vi "Andor_Configuration.vi"(8 "Error in":errorcluster) -> (0 "error out":errorcluster, 3 "image":i32[][](array[numeric]))   [LabVIEW 2011]
uses:
  lib/atmcd32d.llb/ReadMode_mode typedef.ctl
  lib/atmcd32d.llb/AcquisitionMode_mode typedef.ctl
  lib/atmcd32d.llb/TriggerMode_mode typedef.ctl
  lib/atmcd32d.llb/Shutter_type typedef.ctl
  lib/atmcd32d.llb/Shutter_mode typedef.ctl
  lib/atmcd32d.llb/HSSpeed_type typedef.ctl
  lib/atmcd32d.llb/EMGainMode_mode typedef.ctl
  lib/atmcd32d.llb/Error Code Enum typedef.ctl
  Variables/GlobalSetGetConfigureCamera.vi
  Variables/ccdChipPixels.vi
panel:
  out "low":i32
  out "high":i32
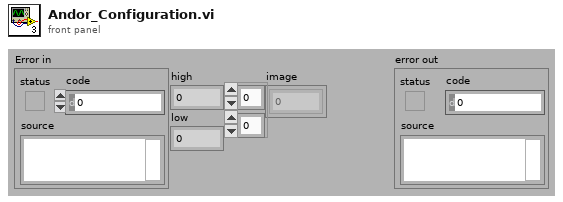
[diagram p1: front panel]
types:
  T1 = typedef "EMGainMode_mode typedef.ctl" = enum16{"8-bit", "12-bit", "Linear", "Real"}
  T2 = typedef "HSSpeed_type typedef.ctl" = enum16{"EM Amp", "Conventional Amp"}
  T3 = typedef "Shutter_mode typedef.ctl" = enum16{"Auto", "Open", "Close"}
  T4 = typedef "Shutter_type typedef.ctl" = enum16{"TTL Low", "TTL High"}
  T5 = typedef "TriggerMode_mode typedef.ctl" = enum16{"Internal", "External", "N/A (2)", "N/A (3)", "N/A (4)", "N/A (5)", "External Start"}
  T6 = typedef "AcquisitionMode_mode typedef.ctl" = enum16{"Reserved (0)", "Single Scan", "Accumulate", "Kinetics", "Fast Kinetics", "Run Till Abort", "Reserved (6)", "Reserved (7)", "Reserved (8)", "Time Delayed Integration"}
  T7 = typedef "ReadMode_mode typedef.ctl" = enum16{"Full Vertical Binning", "Multi-Track", "Random-Track", "Single-Track", "Image"}
  T8 = typedef "Error Code Enum typedef.ctl" = enum32{"N/A (0)", "DRV_ERROR_CODES", "DRV_SUCCESS", "DRV_VXDNOTINSTALLED", "DRV_ERROR_SCAN", "DRV_ERROR_CHECK_SUM", "DRV_ERROR_FILELOAD", "DRV_UNKNOWN_FUNC", "DRV_ERROR_VXD_INIT", "DRV_ERROR_ADDRESS", "DRV_ERROR_PAGELOCK", "DRV_ERROR_PAGEUNLOCK", "DRV_ERROR_BOARDTEST", "DRV_ERROR_ACK", "DRV_ERROR_UP_FIFO", "DRV_ERROR_PATTERN", "N/A (16)", "DRV_ACQUISITION_ERRORS", "DRV_ACQ_BUFFER", "DRV_ACQ_DOWNFIFO_FULL", "DRV_PROC_UNKONWN_INSTRUCTION", "DRV_ILLEGAL_OP_CODE", "DRV_KINETIC_TIME_NOT_MET", "DRV_ACCUM_TIME_NOT_MET", "DRV_NO_NEW_DATA", "N/A (25)", "DRV_SPOOLERROR", "N/A (27)", "N/A (28)", "N/A (29)", "N/A (30)", "N/A (31)", "N/A (32)", "DRV_TEMPERATURE_CODES", "DRV_TEMPERATURE_OFF", "DRV_TEMPERATURE_NOT_STABILIZED", "DRV_TEMPERATURE_STABILIZED", "DRV_TEMPERATURE_NOT_REACHED", "DRV_TEMPERATURE_OUT_RANGE", "DRV_TEMPERATURE_NOT_SUPPORTED", "DRV_TEMPERATURE_DRIFT", "N/A (41)", "N/A (42)", "N/A (43)", "N/A (44)", "N/A (45)", "N/A (46)", "N/A (47)", "N/A (48)", "DRV_GENERAL_ERRORS", "DRV_INVALID_AUX", "DRV_COF_NOTLOADED", "DRV_FPGAPROG", "DRV_FLEXERROR", "DRV_GPIBERROR", "N/A (55)", "N/A (56)", "N/A (57)", "N/A (58)", "N/A (59)", "N/A (60)", "N/A (61)", "N/A (62)", "N/A (63)", "DRV_DATATYPE", "DRV_DRIVER_ERRORS", "DRV_P1INVALID", "DRV_P2INVALID", "DRV_P3INVALID", "DRV_P4INVALID", "DRV_INIERROR", "DRV_COFERROR", "DRV_ACQUIRING", "DRV_IDLE", "DRV_TEMPCYCLE", "DRV_NOT_INITIALIZED", "DRV_P5INVALID", "DRV_P6INVALID", "DRV_INVALID_MODE", "DRV_INVALID_FILTER", "DRV_I2CERRORS", "DRV_I2CDEVNOTFOUND", "DRV_I2CTIMEOUT", "DRV_P7INVALID", "N/A (84)", "N/A (85)", "N/A (86)", "N/A (87)", "N/A (88)", "N/A (89)", "DRV_IOCERROR", "DRV_VRMVERSIONERROR"}
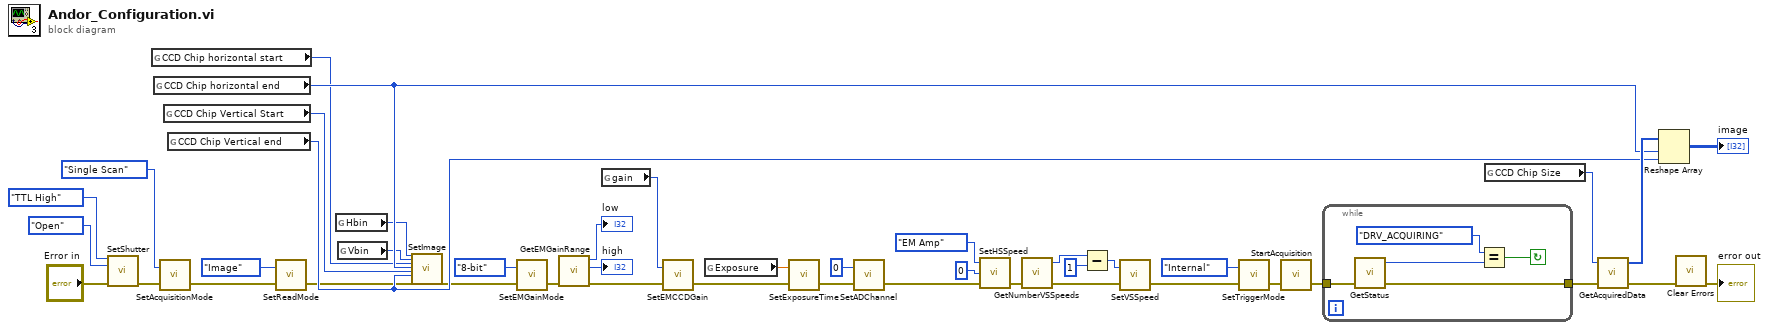
[diagram p0: block diagram]
diagram:
  n1 = call "SetShutter.vi"("type"=Shutter_type_typedef."TTL High", "mode"=Shutter_mode_typedef."Open", "error in (no error)"="Error in") -> ("error out"=w7:errorcluster)  [unwired: 11 in, 1 out]
  n2 = global read "ccdChipPixels.vi" "CCD Chip horizontal start"() -> (w33:i32)
  n3 = global read "ccdChipPixels.vi" "CCD Chip horizontal end"() -> (w41:i32)
  n4 = call "SetAcquisitionMode.vi"("error in (no error)"=w7, "mode"=AcquisitionMode_mode_typedef."Single Scan") -> ("error out"=w31:errorcluster)  [unwired: 1 out]
  n5 = global read "ccdChipPixels.vi" "CCD Chip Vertical Start"() -> (w32:i32)
  n6 = global read "ccdChipPixels.vi" "CCD Chip Vertical end"() -> (w40:i32)
  n7 = call "SetReadMode.vi"("error in (no error)"=w31, "mode"=ReadMode_mode_typedef."Image") -> ("error out"=w30:errorcluster)  [unwired: 1 out]
  n8 = global read "GlobalSetGetConfigureCamera.vi" "Hbin"() -> (w36:i32)
  n9 = global read "GlobalSetGetConfigureCamera.vi" "Vbin"() -> (w37:i32)
  n10 = call "SetImage.vi"("hbin"=w36, "vbin"=w37, "hstart"=w33, "hend"=w41, "vstart"=w32, "vend"=w40, "error in (no error)"=w30) -> ("error out"=w5:errorcluster)  [unwired: 19 in, 1 out]
  n11 = call "SetEMGainMode.vi"("error in (no error)"=w5, "mode"=EMGainMode_mode_typedef."8-bit") -> ("error out"=w11:errorcluster)  [unwired: 1 out]
  n12 = call "GetEMGainRange.vi"("error in (no error)"=w11) -> ("error out"=w10:errorcluster, "high"=→"high":i32, "low"=→"low":i32)  [unwired: 3 in, 1 out]
  n13 = global read "GlobalSetGetConfigureCamera.vi" "gain"() -> (w34:i32)
  n14 = call "SetEMCCDGain.vi"("error in (no error)"=w10, "gain"=w34) -> ("error out"=w12:errorcluster)  [unwired: 1 out]
  n15 = global read "GlobalSetGetConfigureCamera.vi" "Exposure"() -> (w35:sgl)
  n16 = call "SetExposureTime.vi"("error in (no error)"=w12, "time"=w35) -> ("error out"=w29:errorcluster)  [unwired: 1 out]
  n17 = call "SetADChannel.vi"("error in (no error)"=w29, "channel"=0) -> ("error out"=w28:errorcluster)  [unwired: 1 out]
  n18 = call "SetHSSpeed.vi"("error in (no error)"=w28, "index"=0, "type"=HSSpeed_type_typedef."EM Amp") -> ("error out"=w24:errorcluster)  [unwired: 1 in, 1 out]
  n19 = call "GetNumberVSSpeeds.vi"("error in (no error)"=w24) -> ("error out"=w22:errorcluster, "number"=w25:i32)  [unwired: 2 in, 1 out]
  n20 = Subtract(x=w25, y=1) -> (x-y=w27:i32)
  n21 = call "SetVSSpeed.vi"("error in (no error)"=w22, "index"=w27) -> ("error out"=w23:errorcluster)  [unwired: 1 out]
  n22 = call "SetTriggerMode.vi"("error in (no error)"=w23, "mode"=TriggerMode_mode_typedef."Internal") -> ("error out"=w6:errorcluster)  [unwired: 1 out]
  n23 = call "StartAcquisition.vi"("error in (no error)"=w6) -> ("error out"=w3:errorcluster)  [unwired: 1 in, 1 out]
  n24 = while {
    tunnel: w3 -> [w48]
    tunnel: [w47] -> w2
    stop <- w44 continue-if-true
    n25 = call "GetStatus.vi"("error in (no error)"=w48) -> ("error out"=w47:errorcluster, "status"=w45:T8)  [unwired: 2 in, 1 out]
    n26 = Equal?(x=Error_Code_Enum_typedef."DRV_ACQUIRING" ("status"), y=w45) -> (x = y?=w44:bool)
  }
  n27 = global read "ccdChipPixels.vi" "CCD Chip Size"() -> (w4:i32)
  n28 = call "GetAcquiredData.vi"("error in (no error)"=w2, "size"=w4) -> ("error out"=w1:errorcluster, "array"=w42:i32[])  [unwired: 1 in, 1 out]
  n29 = Reshape Array(w42, w41, w40) -> (→"image":i32[][])
  n30 = call <vilib>:"Clear Errors.vi"("error in (no error)"=w1) -> ("error out"=→"error out":errorcluster)  [unwired: 6 in]
